vi "Read Wavelength.vi"(8 "error in (no error)":errorcluster, 11 "Stepper.lvclass in":refnum<class "Stepper.lvclass">) -> (0 "error out":errorcluster, 2 "Current Wavelength":dbl[unit] step=1e-09, 3 "Stepper.lvclass out":refnum<class "Stepper.lvclass">)   [LabVIEW 2023, in "Stepper.lvclass"]
uses:
  Stepper.lvclass
  Stepper.lvclass/Stepper.ctl
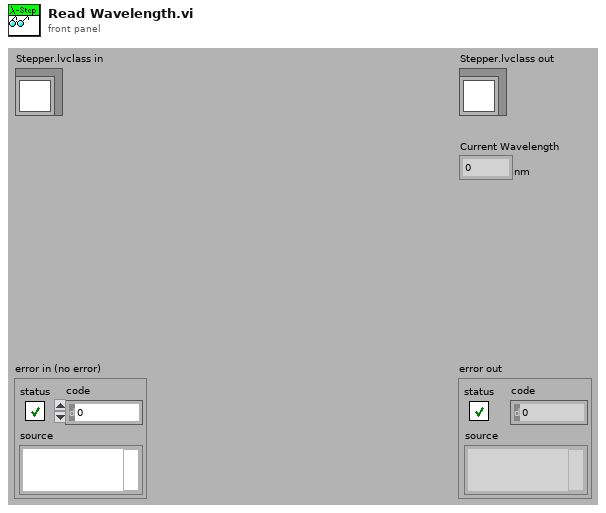
[diagram p1: front panel]
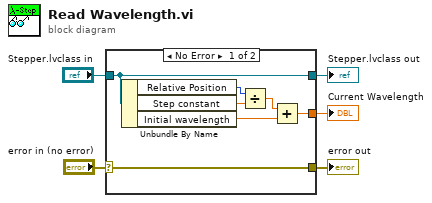
[diagram p0: block diagram]
diagram:
  n1 = case shown="No Error" "error in (no error)" {
    selector: "error in (no error)" -> [w12 w13]
    tunnel: [w12 w13] -> w4
    tunnel: [w11 w14] -> w2
    tunnel: "Stepper.lvclass in" -> [w11 w14]
    tunnel: [w7 _] -> w1
    frame No Error {
      n2 = Unbundle By Name(w11) -> ("Relative Position"=w10:i32, "Step constant"=w9:dbl[unit], "Initial wavelength"=w6:dbl[unit])
      n3 = Divide(x=w10, y=w9) -> (x/y=w8:dbl[unit])
      n4 = Add(x=w8, y=w6) -> (x+y=w7:dbl[unit])
    }
    frame Error {
    }
  }
  "error out" <- w4
  "Stepper.lvclass out" <- w2
  "Current Wavelength" <- w1
